vi "Byte_Generator.vi"(0 "Data_In":T1, 5 "Byte_Array":dbl[](array[numeric])) -> (4 "Data_Out":T1)   [LabVIEW 2021]
doc: "Used to generate the Waveform samples"
uses:
  Controls/Byte_Generator_Data.ctl
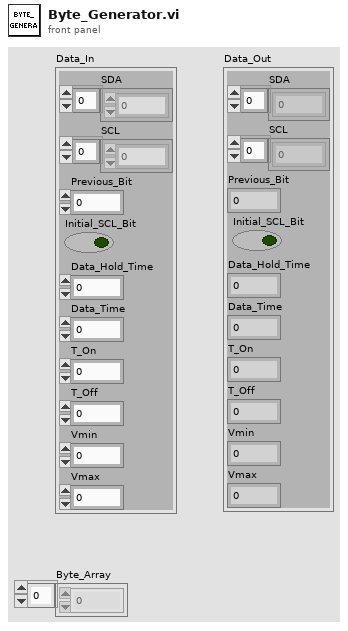
[diagram p1: front panel]
types:
  T1 = typedef "Byte_Generator_Data.ctl" = cluster{"SDA":dbl[], "SCL":dbl[], "Previous_Bit":dbl, "Initial_SCL_Bit":bool, "Data_Hold_Time":i32, "Data_Time":i32, "T_On":i32, "T_Off":i32, "Vmin":dbl, "Vmax":dbl}
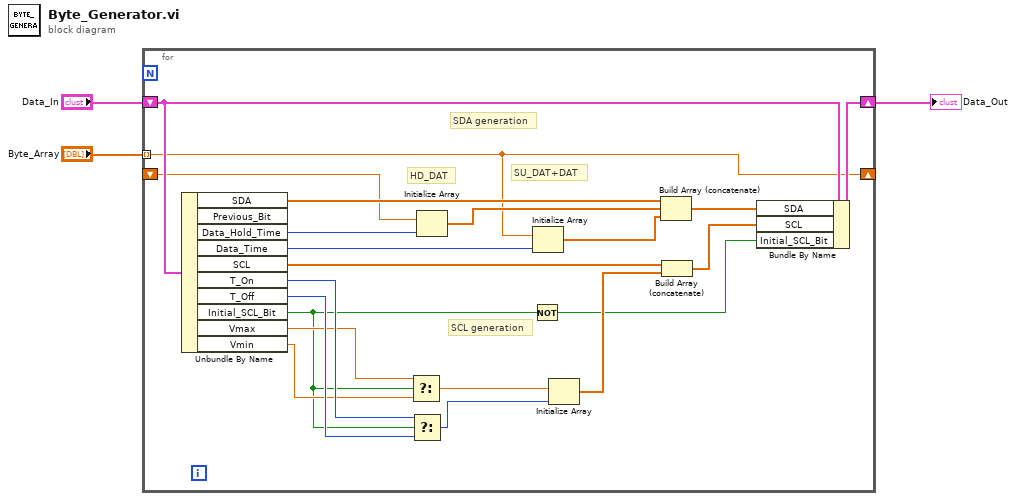
[diagram p0: block diagram]
diagram:
  n1 = for {
    shift-right: [w20] -> w2
    shift-left: "Data_In" -> [w21]
    tunnel: "Byte_Array" -> [w9] mode=indexing
    shift-right: [w9] -> _
    shift-left: _ -> [w8]
    # "HD_DAT"
    # "SDA generation"
    # "SCL generation"
    # "SU_DAT+DAT"
    n2 = Unbundle By Name(w21) -> ("SDA"=w22:dbl[], "Data_Hold_Time"=w14:i32, "Data_Time"=w13:i32, "SCL"=w10:dbl[], "T_On"=w12:i32, "T_Off"=w11:i32, "Initial_SCL_Bit"=w5:bool, "Vmax"=w7:dbl, "Vmin"=w6:dbl)  [unwired: 1 out]
    n3 = Select(t=w7, s=w5, f=w6) -> (s? t:f=w4:dbl)
    n4 = Select(t=w12, s=w5, f=w11) -> (s? t:f=w24:i32)
    n5 = Initialize Array(w8, w14) -> (w15:dbl[])
    n6 = Not(x=w5) -> (.not. x?=w17:bool)
    n7 = Initialize Array(w9, w13) -> (w16:dbl[])
    n8 = Initialize Array(w4, w24) -> (w23:dbl[])
    n9 = Build Array (concatenate)(w22, w15, w16) -> (w19:dbl[])
    n10 = Build Array (concatenate)(w10, w23) -> (w18:dbl[])
    n11 = Bundle By Name(cluster=w21, "SDA"=w19, "SCL"=w18, "Initial_SCL_Bit"=w17) -> (w20:T1)
  }
  "Data_Out" <- w2
